vi "Grab Server Values.vi"(6 "error in (no error)":errorcluster, 8 "Lines":T1[](array[typedef]) {"OPC UA Data Type" items=["Boolean"=1, "SByte"=2, "Byte"=3, "Int16"=4, "UInt16"=5, "Int32"=6, "UInt32"=7, "Int64"=8, "UInt64"=9, "Float"=10, "Double"=11, "String"=12, "DateTime"=13, "ByteString"=15, "Array of Boolean"=101, "Array of SByte"=102, "Array of Byte"=103, "Array of Int16"=104, "Array of UInt16"=105, "Array of Int32"=106, "Array of UInt32"=107, "Array of Int64"=108, "Array of UInt64"=109, "Array of Float"=110, "Array of Double"=111, "Array of String"=112, "Array of DateTime"=113, "Array of ByteString"=115]}, 9 "OPC UA server refnum":refnum<k21>) -> (0 "error out":errorcluster, 2 "Server Data":T3(array[cluster]), 3 "OPC UA server refnum":refnum<k21>)   [LabVIEW 2013, in "OPC UA Client Tests.lvlib"]
uses:
  OPC UA Client Tests.lvlib
  module/configuration/Line.ctl
  <vilib>/NI/Tag Bus Module Framework/channel/TBM channel.lvclass
  module/configuration/OPC UA Data Type.ctl
  module/configuration/OPC UA Client configuration.lvclass
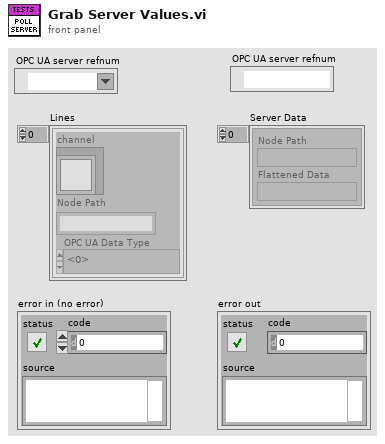
[diagram p1: front panel]
types:
  T1 = typedef "OPC UA Client configuration.lvclass/Line.ctl" = cluster{"channel":refnum<class "TBM channel.lvclass">, "Node Path":string, "OPC UA Data Type":T2}
  T2 = typedef "OPC UA Client configuration.lvclass/OPC UA Data Type.ctl" = u16
  T3 = cluster{"Node Path":string, "Flattened Data":string}[]
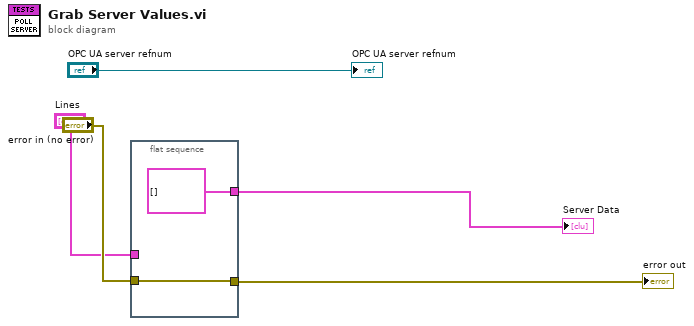
[diagram p0: block diagram]
diagram:
  n1 = flat-sequence {
    tunnel: "Lines" -> [_]
    tunnel: "error in (no error)" -> [w7]
    tunnel: [w7] -> w4
    tunnel: [T3 [] ("Server Data")] -> w5
    frame #0 {
    }
  }
  "Server Data" <- w5
  "error out" <- w4
  "OPC UA server refnum" <- "OPC UA server refnum"
